vi "test_timer.vi"() -> ()   [LabVIEW 2017]
panel:
  out "timeout":bool
  in  "limit s":dbl
  out "time":dbl
  in  "cmd":enum16{"reset", "read"}(ring)
  in  "정지":bool
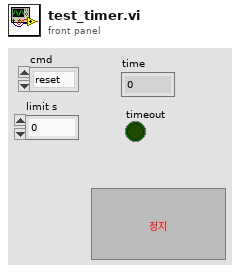
[diagram p1: front panel]
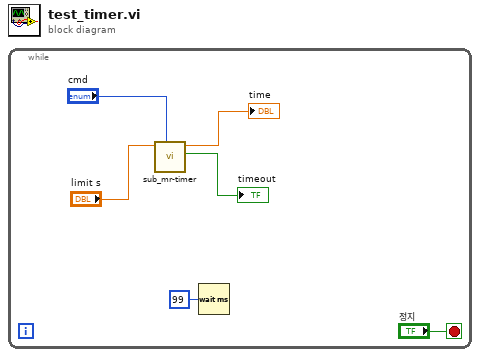
[diagram p0: block diagram]
diagram:
  n1 = while {
    stop <- "정지" stop-if-true
    n2 = call "sub_mr-timer.vi"("cmd"="cmd", "limit s"="limit s") -> ("timeout"=→"timeout":bool, "time"=→"time":dbl)  [unwired: 8 in]
    n3 = Wait (ms)(milliseconds to wait=u32 99 ("대기 시간 (ms)")) -> ()  [unwired: 1 out]
  }
